vi "pic_Limit.vi"(3 "小平台X轴限位":dbl, 4 "小平台X轴当前位置":dbl, 5 "错误输入":errorcluster caption="错误输入（无错误）", 6 "com in":refnum<visa-resource-name>) -> (0 "错误输出":errorcluster, 1 "Limit out":bool[](array[boolean]), 2 "com out":refnum<visa-resource-name>)   [LabVIEW 2018]
panel:
  # "读取IO上的限位"
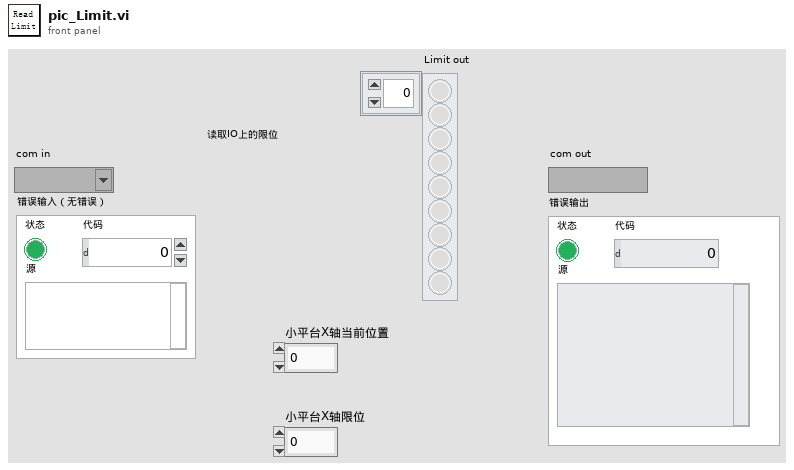
[diagram p1: front panel]
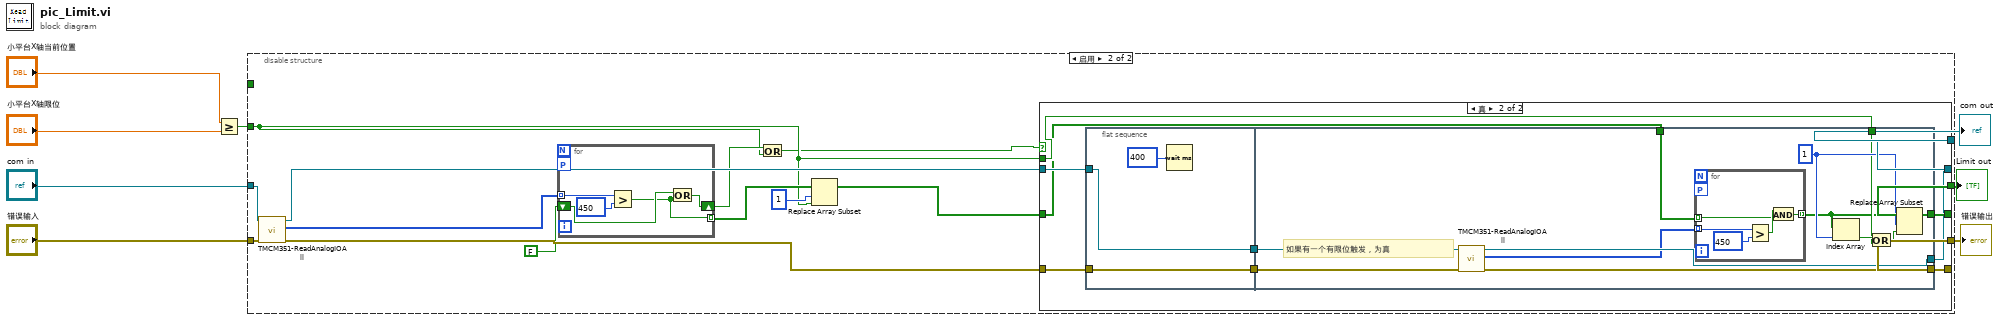
[diagram p0: block diagram]
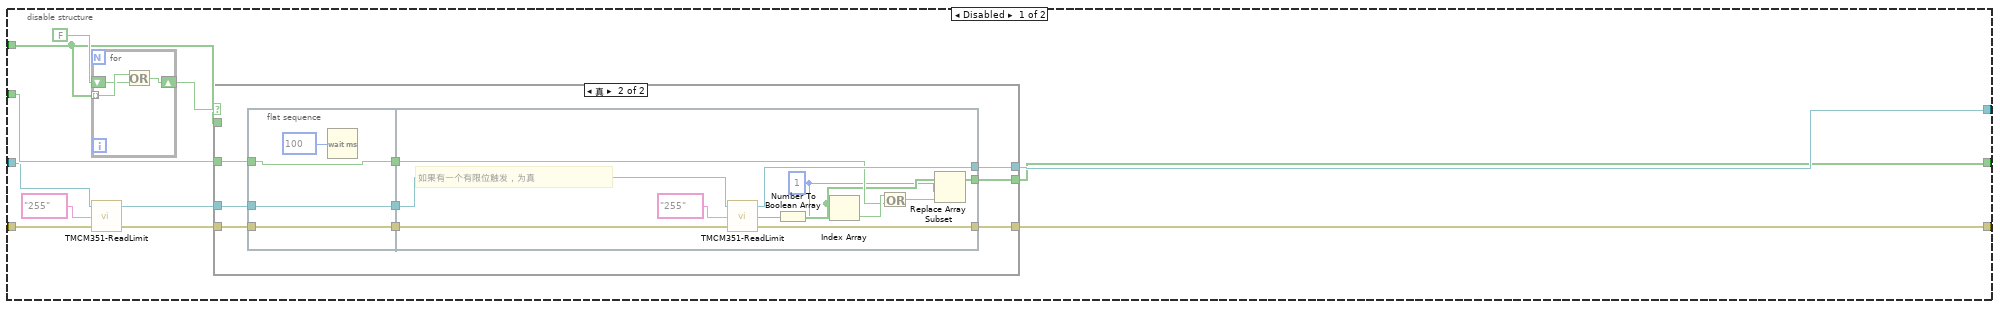
[diagram p2: hidden frame]
diagram:
  n1 = Greater Or Equal?(x="小平台X轴当前位置", y="小平台X轴限位") -> (x >= y?=w4:bool)
  n2 = disable-structure shown="启用" {
    disable-tunnel: [w18 w59] -> w6
    disable-tunnel: [w17 w57] -> w5
    disable-tunnel: w4 -> [w16 w53]
    disable-tunnel: [w15 w58] -> w3
    disable-tunnel: _ -> [w14 _]
    disable-tunnel: "错误输入" -> [w13 w65]
    disable-tunnel: "com in" -> [w11 w66]
    frame Disabled {
      n3 = for {
        tunnel: w14 -> [w51] mode=indexing
        shift-right: [w49] -> w19
        shift-left: FALSE -> [w50]
        n4 = Or(x=w51, y=w50) -> (x .or. y?=w49:bool)
      }
      n5 = call "TMCM351-ReadLimit.vi"("错误输入"=w13, "通道"="255", "com in"=w11) -> ("错误输出"=w10:errorcluster, "com out"=w9:refnum<visa-resource-name>)  [unwired: 1 out]
      n6 = case shown="真" w19 {
        tunnel: w9 -> [w23 w32]
        tunnel: w10 -> [w22 w31]
        tunnel: [w23 w30] -> w18
        tunnel: [w22 w29] -> w17
        tunnel: w16 -> [_ w28]
        tunnel: [w21 w27] -> w15
        tunnel: w14 -> [w21 _]
        frame False {
        }
        frame True {
          n7 = flat-sequence {
            tunnel: w28 -> [w34]
            tunnel: w31 -> [w35]
            tunnel: w32 -> [w36]
            tunnel: [w36] -> w26
            tunnel: [w35] -> w25
            tunnel: [w34] -> w24
            tunnel: [w46] -> w30
            tunnel: [w45] -> w29
            tunnel: [w37] -> w27
            tunnel: w26 -> [w48]
            tunnel: w25 -> [w47]
            tunnel: w24 -> [w41]
            frame #0 {
              n8 = Wait (ms)(milliseconds to wait=u32 100 ("等待时间（毫秒）")) -> ()  [unwired: 1 out]
            }
            frame #1 {
              w38 = 1 ("索引")
              # "如果有一个有限位触发，为真"
              n9 = call "TMCM351-ReadLimit.vi"("错误输入"=w47, "通道"="255", "com in"=w48) -> ("错误输出"=w45:errorcluster, "Dout"=w43:i32, "com out"=w46:refnum<visa-resource-name>)
              n10 = Number To Boolean Array(number=w43) -> (Boolean array=w40:bool[])
              n11 = Index Array(array=w40, index=w38) -> (element=w42:bool)
              n12 = Or(x=w42, y=w41) -> (x .or. y?=w39:bool)
              n13 = Replace Array Subset(array=w40, new element=w39, index=w38) -> (w37:bool[])
            }
          }
        }
      }
    }
    frame Enabled {
      n14 = call "TMCM351-ReadAnalogIOAll.vi"("错误输入"=w65, "com in"=w66) -> ("错误输出"=w60:errorcluster, "AnalogOut"=w64:i32[], "comOut"=w61:refnum<visa-resource-name>)  [unwired: 3 in]
      n15 = for {
        tunnel: w64 -> [w103] mode=indexing
        tunnel: [w100] -> w63 mode=indexing
        workers-P: _ -> [_]
        shift-right: [w99] -> w54
        shift-left: FALSE -> [w101]
        n16 = Greater?(x=w103, y=450) -> (0:w100:bool)
        n17 = Or(x=w101, y=w100) -> (x .or. y?=w99:bool)
      }
      n18 = Or(x=w54, y=w53) -> (x .or. y?=w52:bool)
      n19 = Replace Array Subset(array=w63, new element=w53, index=1 ("索引")) -> (w56:bool[])
      n20 = case shown="真" w52 {
        tunnel: w61 -> [w69 w78]
        tunnel: w60 -> [w68 w77]
        tunnel: [w69 w72] -> w59
        tunnel: [w68 w71] -> w57
        tunnel: [w67 w76] -> w58
        tunnel: w53 -> [_ w73]
        tunnel: w56 -> [w67 w70]
        frame False {
        }
        frame True {
          n21 = flat-sequence {
            tunnel: w77 -> [w80]
            tunnel: w78 -> [w81]
            tunnel: [w81] -> w75
            tunnel: [w80] -> w74
            tunnel: [w90] -> w76
            tunnel: w75 -> [w88]
            tunnel: w74 -> [w87]
            tunnel: w73 -> [w89]
            tunnel: [w86] -> w72
            tunnel: [w85] -> w71
            tunnel: w70 -> [w83]
            frame #0 {
              n22 = Wait (ms)(milliseconds to wait=u32 400 ("等待时间（毫秒）")) -> ()  [unwired: 1 out]
            }
            frame #1 {
              w91 = 1 ("索引")
              # "如果有一个有限位触发，为真"
              n23 = call "TMCM351-ReadAnalogIOAll.vi"("错误输入"=w87, "com in"=w88) -> ("错误输出"=w85:errorcluster, "AnalogOut"=w84:i32[], "comOut"=w86:refnum<visa-resource-name>)  [unwired: 3 in]
              n24 = for {
                tunnel: w84 -> [w98] mode=indexing
                workers-P: _ -> [_]
                tunnel: w83 -> [w95] mode=indexing
                tunnel: [w94] -> w82 mode=indexing
                n25 = Greater?(x=w98, y=450) -> (0:w96:bool)
                n26 = And(x=w96, y=w95) -> (x .and. y?=w94:bool)
              }
              n27 = Index Array(array=w82, index=w91) -> (element=w93:bool)
              n28 = Or(x=w93, y=w89) -> (x .or. y?=w92:bool)
              n29 = Replace Array Subset(array=w82, new element=w92, index=w91) -> (w90:bool[])
            }
          }
        }
      }
    }
  }
  "com out" <- w6
  "错误输出" <- w5
  "Limit out" <- w3
